vi "checkpoint test 1.vi"() -> ()   [LabVIEW 2009]
uses:
  object.ctl
  <vilib>/Utility/miscctls.llb/LVPositionTypeDef.ctl
  <vilib>/Utility/miscctls.llb/LVPointTypeDef.ctl
panel:
  in  "Tab":enum32{"draw", "test", "stop"}(tab)
  in  "checkpoint?":bool
  in  "clear picture":bool
  in  "weight":dbl(slide) min=-10.0 max=10.0 step=0.5 scale=-10.0..10.0
  in  "start point":cluster{"x":i16, "y":i16}
  in  "Speed":sgl(slide) scale=0.0..10.0
  in  "milliseconds to wait":u32(slide) scale=10.0..1000.0
  out "location":cluster{i16, i16}
  in  "Array":T1[](array[typedef])
  out "Pic":picture
  # "freezing up\nwhen queue is empty"
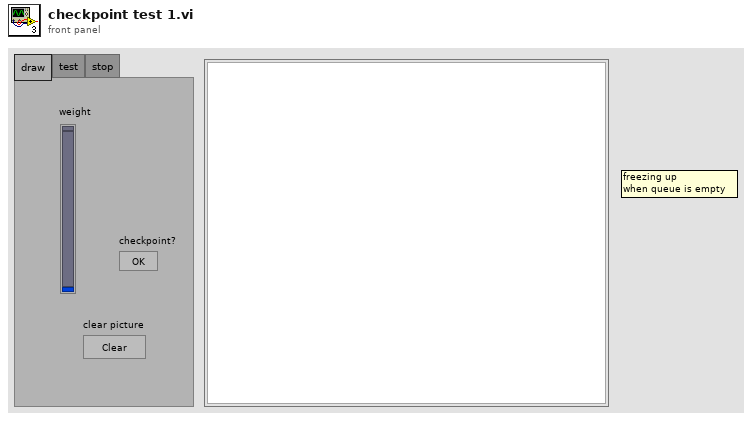
[diagram p1: front panel]
types:
  T1 = typedef "object.ctl" = cluster{"rect":cluster{"left":i16, "top":i16, "right":i16, "bottom":i16}, "weight":sgl}
  T2 = typedef "LVPointTypeDef.ctl" = cluster{"Horizontal":i16, "Vertical":i16}
  T3 = typedef "LVPositionTypeDef.ctl" = cluster{"Left":i32, "Top":i32}
  T4 = cluster{"left":i16, "top":i16, "right":i16, "bottom":i16}
  T5 = typedef "LVPoint32TypeDef.ctl" = cluster{"Horizontal":i32, "Vertical":i32}
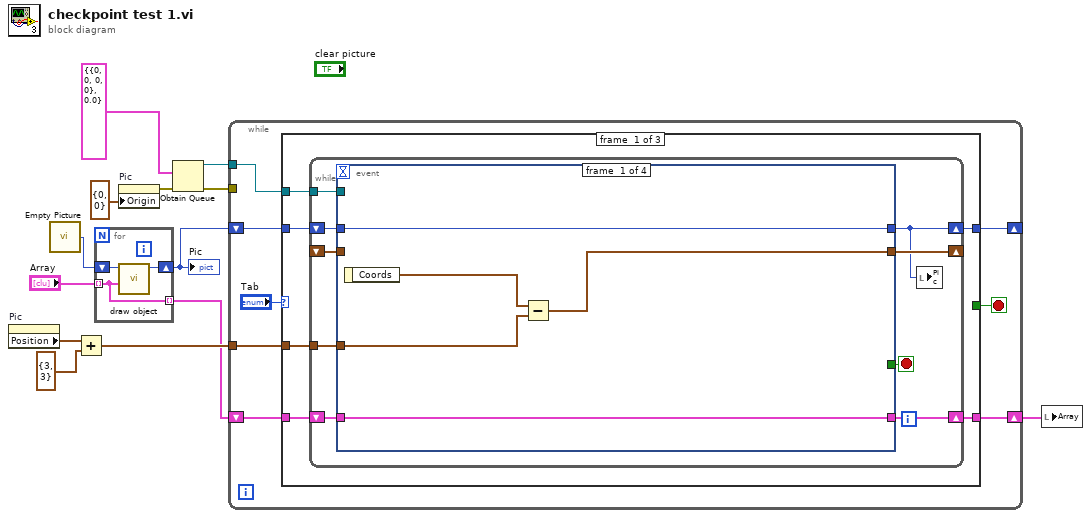
[diagram p0: block diagram]
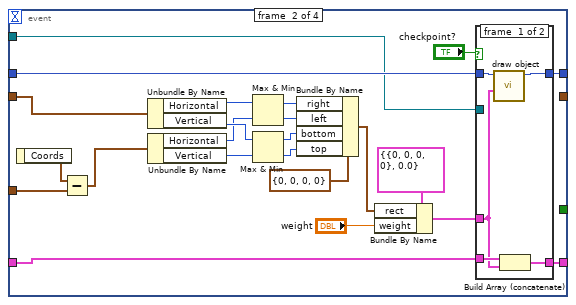
[diagram p2: hidden frame]
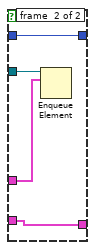
[diagram p3: hidden frame]
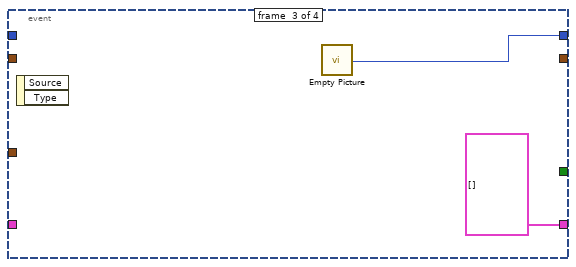
[diagram p4: hidden frame]
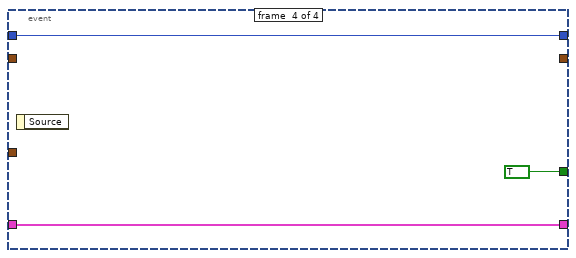
[diagram p5: hidden frame]
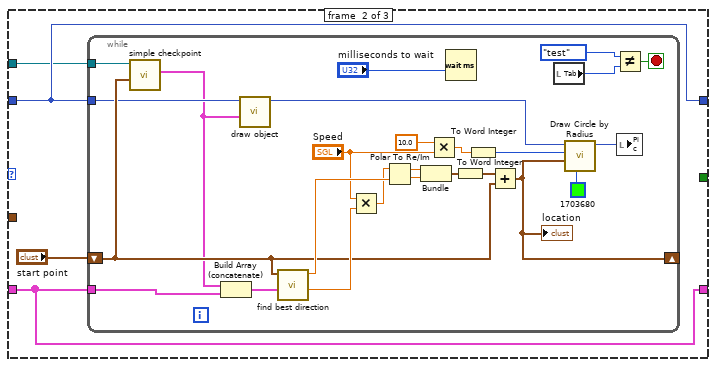
[diagram p6: hidden frame]
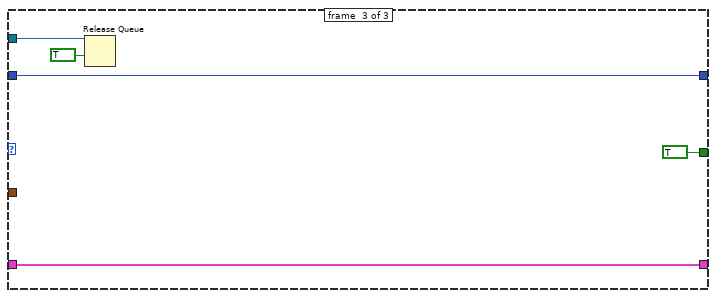
[diagram p7: hidden frame]
diagram:
  n1 = property on="Pic" class="Pict"() -> ("Position"=w13:T3)  [unwired: 2 in, 2 out]
  n2 = call "Empty Picture"() -> ("empty picture"=w6:picture)
  n3 = Add(x=w13, y=T3 {"Left"=3, "Top"=3}) -> (x+y=w11:T3)
  n4 = for {
    tunnel: "Array" -> [w14] mode=indexing
    shift-right: [w16] -> w5
    shift-left: w6 -> [w15]
    tunnel: [w14] -> w7 mode=indexing
    n5 = call "draw object.vi"("Object"=w14, "picture in"=w15) -> ("picture out"=w16:picture)  [unwired: 9 in]
  }
  "Pic" <- w5
  n6 = property on="Pic" class="Pict"("Origin"=T2 {"Horizontal"=0, "Vertical"=0}) -> (error out=w4:errorcluster)  [unwired: 2 in, 1 out]
  n7 = Obtain Queue(element data type=T1 {"rect"={"left"=0, "top"=0, "right"=0, "bottom"=0}, "weight"=0.0} ("Object"), error in (no error)=w4) -> (queue out=w2:refnum<queue>, error out=w3:errorcluster)  [unwired: 3 in, 1 out]
  n8 = while {
    shift-right: [w24] -> _
    shift-left: w5 -> [w23]
    shift-right: [w20] -> w9
    shift-left: w7 -> [w21]
    tunnel: w11 -> [w18]
    tunnel: w3 -> [_]
    tunnel: w2 -> [w17]
    stop <- w19 stop-if-true
    n9 = case shown="\"test\"" "Tab" {
      tunnel: [w30 w85 w115] -> w24
      tunnel: w23 -> [w29 w85 w115]
      tunnel: w21 -> [w28 w84 w114]
      tunnel: [w27 w84 w114] -> w20
      tunnel: [_ _ TRUE] -> w19
      tunnel: w18 -> [w26 _ _]
      tunnel: w17 -> [w25 w82 w112]
      frame #0 {
        n10 = while {
          shift-right: [w39] -> _
          shift-left: _ -> [w38]
          shift-right: [w33] -> w30
          shift-left: w29 -> [w37]
          shift-right: [w34] -> w27
          shift-left: w28 -> [w35]
          tunnel: w26 -> [w32]
          tunnel: w25 -> [w31]
          stop <- w36 stop-if-true
          n11 = event shown="[1] \"Pic\": Mouse Up" {
            selector: _ -> [_ _ _ _]
            dyn-events: _ -> [_ _ _ _]
            timeout: _ -> [_ _ _ _]
            tunnel: [w40 _ _ _] -> w39
            tunnel: w38 -> [_ w67 _ _]
            tunnel: [w44 w53 w77 w79] -> w33
            tunnel: w37 -> [w44 w54 _ w79]
            tunnel: [_ _ _ TRUE] -> w36
            tunnel: w35 -> [w43 w57 _ w80]
            tunnel: [w43 w58 T1[] [] w80] -> w34
            tunnel: w32 -> [w41 w50 _ _]
            tunnel: w31 -> [_ w45 _ _]
            event #0 {
              n12 = event-data() -> ("Coords"=w42:T5)  [unwired: 1 in]
              n13 = Subtract(x=w42, y=w41) -> (x-y=w40:T5)
            }
            event #1 {
              n14 = event-data() -> ("Coords"=w51:T5)  [unwired: 1 in]
              n15 = Subtract(x=w51, y=w50) -> (x-y=w47:T5)
              n16 = Unbundle By Name(w67) -> ("Horizontal"=w66:i32, "Vertical"=w65:i32)
              n17 = Unbundle By Name(w47) -> ("Horizontal"=w48:i32, "Vertical"=w49:i32)
              n18 = Max & Min(x=w66, y=w48) -> (max(x,y)=w60:i32, min(x,y)=w61:i32)
              n19 = Max & Min(x=w65, y=w49) -> (max(x,y)=w63:i32, min(x,y)=w62:i32)
              n20 = Bundle By Name(cluster=T4 {"left"=0, "top"=0, "right"=0, "bottom"=0} ("rect"), "right"=w60, "left"=w61, "bottom"=w63, "top"=w62) -> (w59:T4)
              n21 = Bundle By Name(cluster=T1 {"rect"={"left"=0, "top"=0, "right"=0, "bottom"=0}, "weight"=0.0} ("Object"), "rect"=w59, "weight"="weight") -> (w52:T1)
              n22 = case shown="True" "checkpoint?" {
                tunnel: [w72 w76] -> w58
                tunnel: w57 -> [w71 w76]
                tunnel: w54 -> [w70 w75]
                tunnel: [w69 w75] -> w53
                tunnel: w52 -> [w68 w73]
                tunnel: w45 -> [_ w74]
                frame #0 {
                  n23 = call "draw object.vi"("Object"=w68, "picture in"=w70) -> ("picture out"=w69:picture)  [unwired: 9 in]
                  n24 = Build Array (concatenate)(w71, w68) -> (w72:T1[])
                }
                frame #1 {
                  n25 = Enqueue Element(queue=w74, element=w73) -> ()  [unwired: 2 in, 3 out]
                }
              }
            }
            event #2 {
              n26 = event-data() -> ()  [unwired: 1 in, 2 out]
              n27 = call "Empty Picture"() -> ("empty picture"=w77:picture)
            }
            event #3 {
              n28 = event-data() -> ()  [unwired: 1 in, 1 out]
            }
          }
          n29 = local write "Pic"(w33) -> ()
        }
      }
      frame #1 {
        n30 = while {
          shift-right: [w104] -> _
          shift-left: "start point" -> [w93]
          tunnel: w84 -> [w90]
          tunnel: w85 -> [w92]
          tunnel: w82 -> [w94]
          stop <- w101 stop-if-true
          n31 = call "simple checkpoint.vi"("Current location"=w93, "checkpoint queue"=w94) -> ("next checkpoint"=w88:T1)  [unwired: 9 in]
          n32 = Build Array (concatenate)(w88, w90) -> (w89:T1[])
          n33 = call "draw object.vi"("Object"=w88, "picture in"=w92) -> ("picture out"=w91:picture)  [unwired: 9 in]
          n34 = call "find best direction.vi"("Objects"=w89, "current location"=w93) -> ("magnitude"=w96:sgl, "Direction"=w98:sgl)  [unwired: 8 in]
          n35 = Multiply(x="Speed", y=w96) -> (x*y=w95:sgl)
          n36 = Polar To Re/Im(2:w98, 3:w95) -> (0:w109:sgl, 1:w108:sgl)
          n37 = Bundle(w108, w109) -> (w107:cluster{sgl, sgl})  [unwired: 1 in]
          n38 = Multiply(x=sgl 10.0, y="Speed") -> (x*y=w100:sgl)
          n39 = Wait (ms)(milliseconds to wait="milliseconds to wait") -> ()  [unwired: 1 out]
          n40 = To Word Integer(number=w107) -> (16bit integer=w87:cluster{i16, i16})
          n41 = To Word Integer(number=w100) -> (16bit integer=w103:i16)
          n42 = Add(x=w87, y=w93) -> (x+y=w104:cluster{i16, i16})
          "location" <- w104
          n43 = local read "Tab"() -> (w110:enum32{"draw", "test", "stop"})
          n44 = call <vilib>:"Draw Circle by Radius.vi"("color(black)"=u32 1703680, "pixel center"=w104, "radius"=w103, "picture"=w91) -> ("new picture"=w102:picture)  [unwired: 7 in]
          n45 = Not Equal?(x=enum32{"draw", "test", "stop"}."test" ("Tab"), y=w110) -> (x != y?=w101:bool)
          n46 = local write "Pic"(w102) -> ()
        }
      }
      frame #2 {
        n47 = Release Queue(queue=w112, force destroy? (F)=TRUE) -> ()  [unwired: 1 in, 3 out]
      }
    }
  }
  n48 = local write "Array"(w9) -> ()
